vi "Updater.vi"(8 "error in (no error)":errorcluster) -> (0 "error out":errorcluster, 1 "appended path":path, 2 "return code":i32, 3 "Updating?":bool)   [LabVIEW 2013]
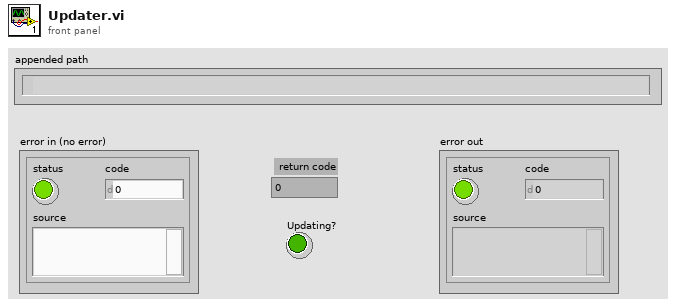
[diagram p1: front panel]
types:
  T1 = enum32{"invalid app kind", "Development System", "Run Time System", "Student Edition", "Embedded LabVIEW", "Evaluation", "Custom"}
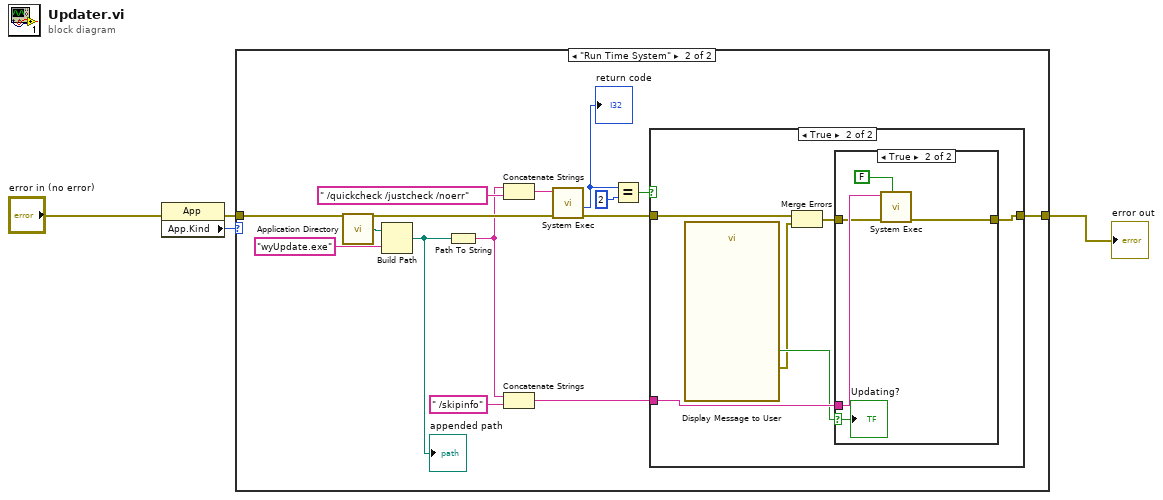
[diagram p0: block diagram]
diagram:
  n1 = property class="App"(error in="error in (no error)") -> (error out=w3:errorcluster, "App.Kind"=w4:T1)  [unwired: 1 in, 1 out]
  n2 = case shown="\"Run Time System\"" w4 {
    tunnel: w3 -> [w5 w19]
    tunnel: [w5 w6] -> w2
    frame "Development System", Default {
    }
    frame "Run Time System" {
      n3 = call <vilib>:"Application Directory.vi"() -> ("Application Directory"=w14:path)
      n4 = Build Path(base path=w14, name or relative path="wyUpdate.exe" ("standard input")) -> (appended path=w17:path)
      "appended path" <- w17
      n5 = Path To String(path=w17) -> (string=w9:string)
      n6 = Concatenate Strings(w9, " /quickcheck /justcheck /noerr" ("standard input")) -> (w15:string)
      n7 = Concatenate Strings(w9, " /skipinfo" ("standard input")) -> (w7:string)
      n8 = call <vilib>:"System Exec.vi"("error in (no error)"=w19, "command line"=w15) -> ("error out"=w10:errorcluster, "return code"=w13:i32)  [unwired: 6 in, 2 out]
      "return code" <- w13
      n9 = Equal?(x=w13, y=2) -> (x = y?=w11:bool)
      n10 = case shown="True" w11 {
        tunnel: w10 -> [w20 w22]
        tunnel: w7 -> [_ w26]
        tunnel: [w20 w25] -> w6
        frame False {
        }
        frame True {
          n11 = call "Display Message to User"() -> ("error out"=w23:errorcluster, "OK"=w24:bool)  [unwired: 10 in]
          n12 = Merge Errors(w22, w23) -> (w21:errorcluster)
          n13 = case shown="True" w24 {
            selector: w24 -> [_ w29]
            tunnel: w26 -> [_ w32]
            tunnel: w21 -> [w27 w31]
            tunnel: [w27 w28] -> w25
            frame False {
            }
            frame True {
              n14 = call <vilib>:"System Exec.vi"("wait until completion? (T)"=FALSE, "error in (no error)"=w31, "command line"=w32) -> ("error out"=w28:errorcluster)  [unwired: 5 in, 3 out]
              "Updating?" <- w29
            }
          }
        }
      }
    }
  }
  "error out" <- w2
